vi "FGV Testdaten sammeln.vi"(0 "Ergebnisse Dichtheitstest":T6 {"Druck FT-IR:" format="%.3f"}, 1 "Kalenderauswertung":string[](array[string]), 5 "Ergebnis T90":T3 {"Leitungslänge" format="%#_5g"; "Rise Time" format="%#.1g"; "T90:" format="%#.1g"; "T50:" format="%#.2g"; "T10:" format="%#.2g"}, 7 "Ergebnisse Kalibrieren":T2, 9 "Ergebnis CalGas Test":T1, 11 "error in (no error)":errorcluster caption="Fehler (Eingang, kein Fehler)", 13 "Aktion":T7) -> (3 "Kalenderauswertung":string[](array[string]), 4 "Ergebnisse Dichtheitstest":T6 {"Druck FT-IR:" format="%.3f"}, 6 "Ergebnis T90":T3 {"Leitungslänge" format="%#_5g"; "Rise Time" format="%#.1g"; "T90:" format="%#.1g"; "T50:" format="%#.2g"; "T10:" format="%#.2g"}, 8 "Ergebnisse Kalibrieren":T2, 10 "Ergebnis CalGas Test":T1, 15 "error out":errorcluster caption="Fehler (Ausgang)")   [LabVIEW 2020, in "Schedule Modul.lvlib"]
uses:
  Schedule Modul.lvlib
  Aktion FGV Testdaten sammeln.ctl
  Ergebnis Dichtheitstest.ctl
  Visualisierungs Elemente/Zahlen-Ausgabefeld.ctl
  Ergebnis Kalibrieren.ctl
  Ergebnis T90.ctl
  Visualisierungs Elemente/Zahlen-Eingabefeld.ctl
  Ergebnis CalGas Test.ctl
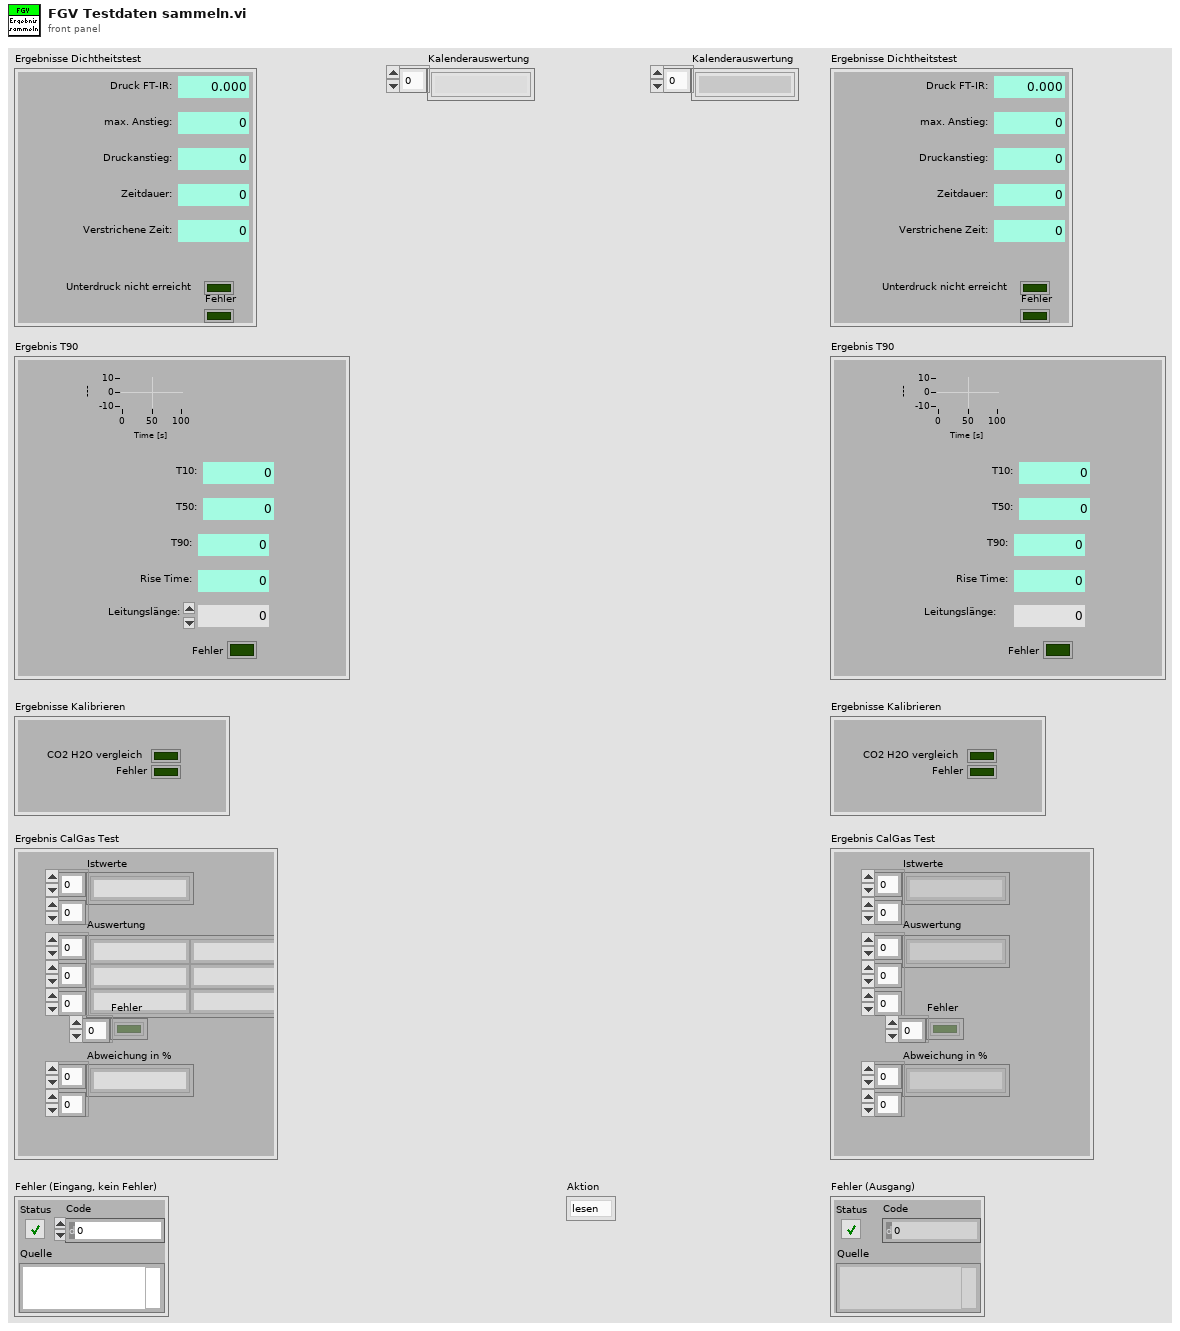
[diagram p1: front panel]
types:
  T1 = typedef "Schedule Modul.lvlib/Ergebnis CalGas Test.ctl" = cluster{"Istwerte":string[][], "Auswertung":string[][][], "Fehler":bool[], "Abweichung in %":string[][]}
  T2 = typedef "Schedule Modul.lvlib/Ergebnis Kalibrieren.ctl" = cluster{"Fehler":bool, "CO2 H2O vergleich":bool}
  T3 = typedef "Schedule Modul.lvlib/Ergebnis T90.ctl" = cluster{"T90":waveform(sgl), "T10:":T4, "T50:":T4, "T90:":T4, "Rise Time":T4, "Leitungslänge":T5, "Fehler":bool}
  T4 = typedef "Zahlen-Ausgabefeld.ctl" = sgl
  T5 = typedef "Zahlen-Eingabefeld.ctl" = sgl
  T6 = typedef "Schedule Modul.lvlib/Ergebnis Dichtheitstest.ctl" = cluster{"Druck FT-IR:":T4, "max. Anstieg:":T4, "Druckanstieg:":T4, "Zeitdauer:":T4, "Verstrichene Zeit:":T4, "Fehler":bool, "Unterdruck nicht erreicht ":bool}
  T7 = typedef "Schedule Modul.lvlib/Aktion FGV Testdaten sammeln.ctl" = enum16{"lesen", "Dichtheitstest", "CalGasTest", "T90", "Kalibrieren", "init", "Kalender Daten"}
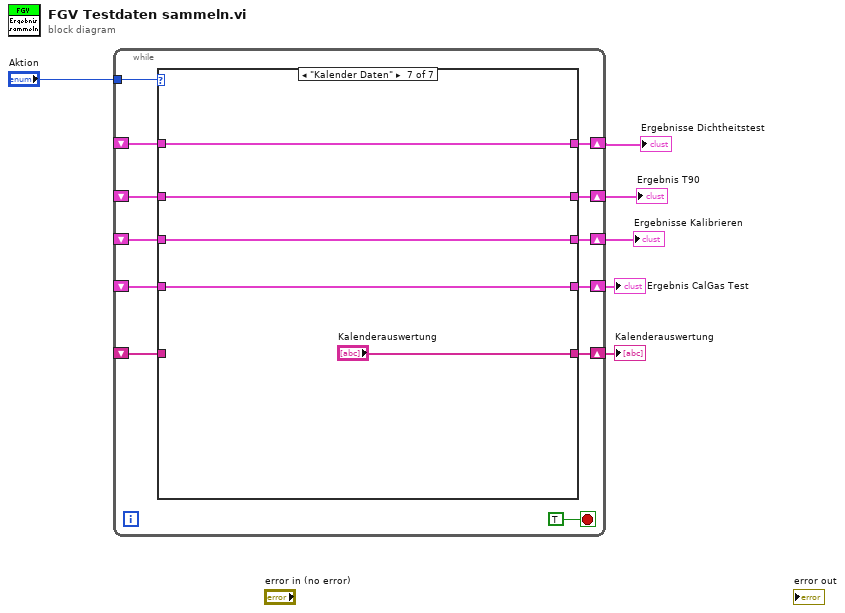
[diagram p0: block diagram]
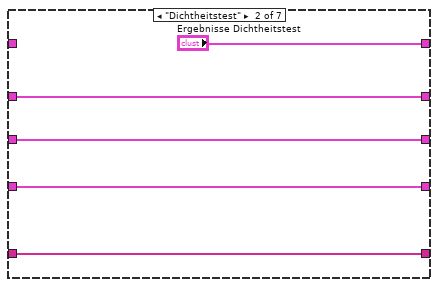
[diagram p3: hidden frame]
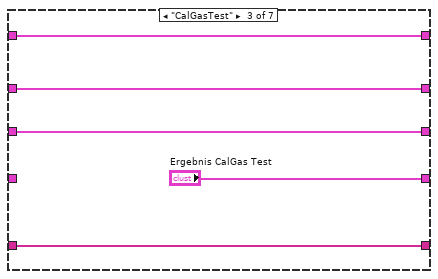
[diagram p4: hidden frame]
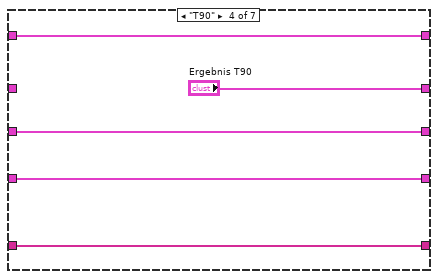
[diagram p5: hidden frame]
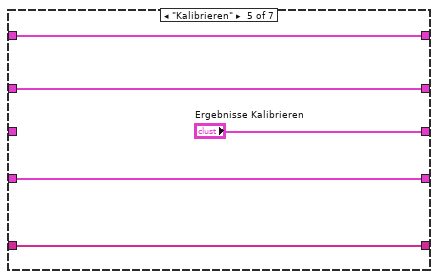
[diagram p6: hidden frame]
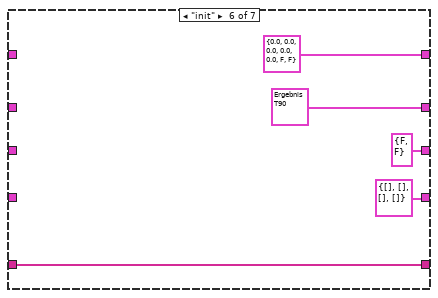
[diagram p7: hidden frame]
diagram:
  n1 = while {
    tunnel: "Aktion" -> [w17]
    shift-right: [w16] -> w5
    shift-left: _ -> [w15]
    shift-right: [w14] -> w4
    shift-left: _ -> [w13]
    shift-right: [w12] -> w3
    shift-left: _ -> [w11]
    shift-right: [w10] -> w2
    shift-left: _ -> [w9]
    shift-right: [w8] -> w1
    shift-left: _ -> [w7]
    stop <- TRUE stop-if-true
    n2 = case shown="\"Kalender Daten\"" w17 {
      tunnel: [w23 "Ergebnisse Dichtheitstest" w33 w38 w43 T6 {"Druck FT-IR:"=0.0, "max. Anstieg:"=0.0, "Druckanstieg:"=0.0, "Zeitdauer:"=0.0, "Verstrichene Zeit:"=0.0, "Fehler"=FALSE, "Unterdruck nicht erreicht "=FALSE} ("Ergebnisse Dichtheitstest") w53] -> w16
      tunnel: w15 -> [w23 _ w33 w38 w43 _ w53]
      tunnel: [w22 w27 w32 "Ergebnis T90" w42 T3 {"T90"={"t0"=timestamp(0 s since 1904-01-01), "dt"=1.0, "Y"=[]}, "T10:"=0.0, "T50:"=0.0, "T90:"=0.0, "Rise Time"=0.0, "Leitungslänge"=0.0, "Fehler"=FALSE} ("Ergebnis T90") w52] -> w14
      tunnel: w13 -> [w22 w27 w32 _ w42 _ w52]
      tunnel: [w21 w26 w31 w36 "Ergebnisse Kalibrieren" T2 {"Fehler"=FALSE, "CO2 H2O vergleich"=FALSE} ("Ergebnisse Kalibrieren") w51] -> w12
      tunnel: w11 -> [w21 w26 w31 w36 _ _ w51]
      tunnel: [w20 w25 "Ergebnis CalGas Test" w35 w40 T1 {"Istwerte"=[], "Auswertung"=[], "Fehler"=[], "Abweichung in %"=[]} ("Ergebnis CalGas Test") w50] -> w10
      tunnel: w9 -> [w20 w25 _ w35 w40 _ w50]
      tunnel: [w19 w24 w29 w34 w39 w44 "Kalenderauswertung"] -> w8
      tunnel: w7 -> [w19 w24 w29 w34 w39 w44 _]
      frame "lesen", Default {
      }
      frame "Dichtheitstest" {
      }
      frame "CalGasTest" {
      }
      frame "T90" {
      }
      frame "Kalibrieren" {
      }
      frame "init" {
      }
      frame "Kalender Daten" {
      }
    }
  }
  "Ergebnis T90" <- w4
  "Ergebnisse Kalibrieren" <- w3
  "Ergebnisse Dichtheitstest" <- w5
  "Ergebnis CalGas Test" <- w2
  "Kalenderauswertung" <- w1
